vi "SciShutter.vi"(7 "Operational Mode":T1, 8 "error in (no error)":errorcluster, 11 "Science":T2={"Time Stamp Control"=timestamp(0 s since 1904-01-01), "State"=FALSE, "Set"=enum."Arm"}) -> (0 "error out":errorcluster={"status"=FALSE, "code"=180121602, "source"="Shared Variable in SciShutter.vi->MainRT.vi<APPEND>\nThis error or warning occurred while reading the following Shared Variable:\n\\\\.\\RT-Variables\\Dummy Trigger\n\\\\.\\RT-Variables\\Dummy Trigger"}, 3 "Science out":T2, 5 "Operational Mode out":T1)   [LabVIEW 2016]
uses:
  Controls/Shutter Data.ctl
  Controls/Shutter States.ctl
  Controls/Operational Modes.ctl
panel:
  in  "Wait time [s]":dbl=0.1 format="%#_13g"
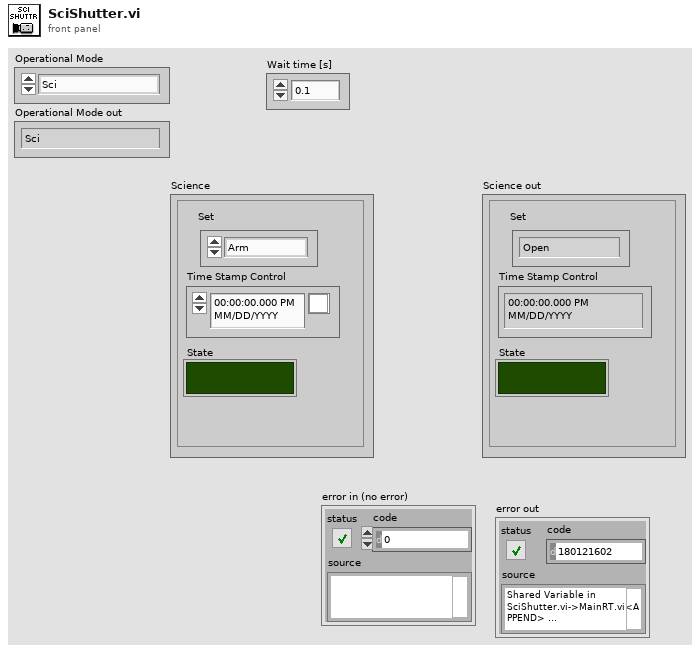
[diagram p1: front panel]
types:
  T1 = typedef "Operational Modes.ctl" = enum16{"Sci", "Sci-LFC", "Solar", "Solar-LFC", "LFC", "LFC-Sim", "LFC-Both", "ThAr", "ThAr-LFC", "Flat", "ExtFlat", "ExtFlat-Sim", "ExtFlat-Both", "Qtz", "ExtQtz", "ExtQtz-Sim", "ExtQtz-Both", "Dark", "Manual", "Off"}
  T2 = typedef "Shutter Data.ctl" = cluster{"Time Stamp Control":timestamp, "State":bool, "Set":T3}
  T3 = typedef "Shutter States.ctl" = enum16{"Open", "Close", "Wait", "Off", "Arm", "Idle"}
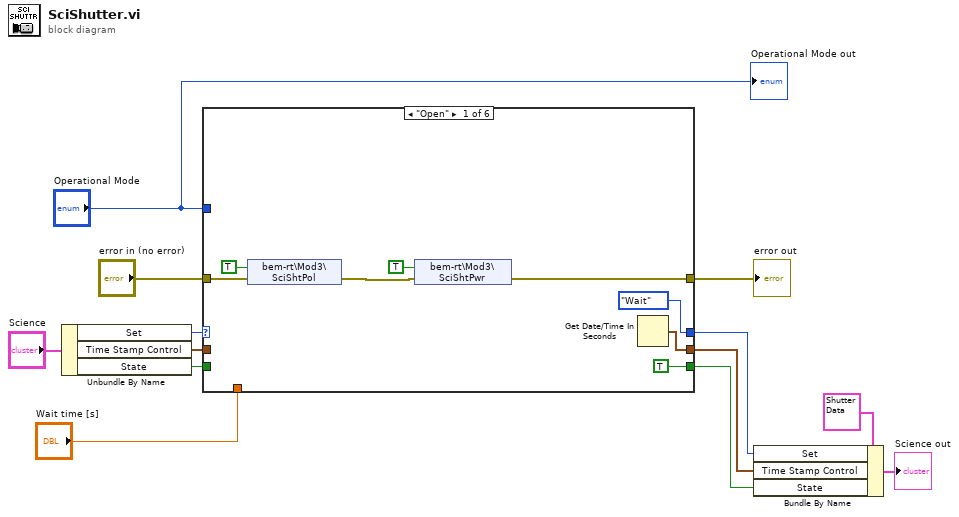
[diagram p0: block diagram]
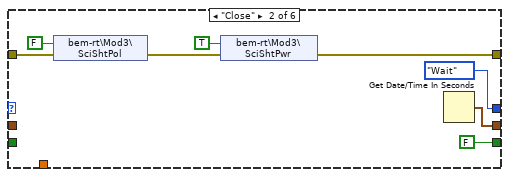
[diagram p2: hidden frame]
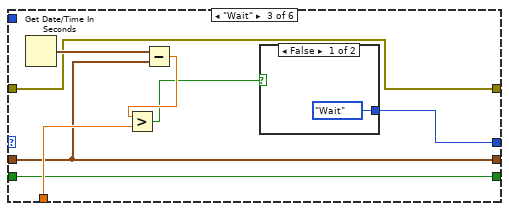
[diagram p3: hidden frame]
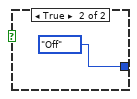
[diagram p4: hidden frame]
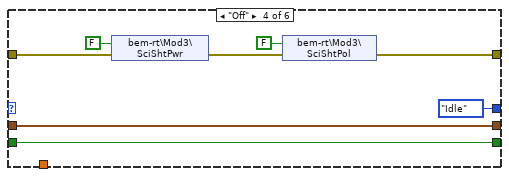
[diagram p5: hidden frame]
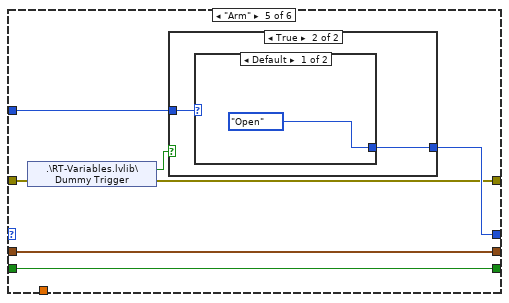
[diagram p6: hidden frame]
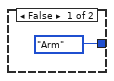
[diagram p7: hidden frame]
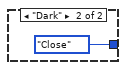
[diagram p8: hidden frame]
diagram:
  n1 = Unbundle By Name("Science") -> ("Set"=w13:T3, "Time Stamp Control"=w11:timestamp, "State"=w9:bool)
  n2 = case shown="\"Open\"" w13 {
    selector: w13 -> [_ _ _ _ _ w63]
    tunnel: [Shutter_States."Wait" ("Set") Shutter_States."Wait" ("Set") w33 Shutter_States."Idle" ("Set") w53 w63] -> w4
    tunnel: w11 -> [_ _ w32 w41 w49 w62]
    tunnel: [w21 w26 w32 w41 w49 w62] -> w10
    tunnel: w9 -> [_ _ w31 w40 w52 w61]
    tunnel: [TRUE ("State") FALSE ("State") w31 w40 w52 w61] -> w8
    tunnel: [w19 w28 w30 w43 w51 w60] -> w7
    tunnel: "error in (no error)" -> [w18 w27 w30 w45 w50 w60]
    tunnel: "Wait time [s]" -> [_ _ w35 _ _ _]
    tunnel: "Operational Mode" -> [_ _ _ _ w48 _]
    frame "Open" {
      n3 = shared-variable "bem-rt\\Mod3\\SciShtPol"(TRUE ("SciShtPol"), error in=w18) -> (error out=w17:errorcluster)
      n4 = shared-variable "bem-rt\\Mod3\\SciShtPwr"(TRUE ("SciShtPwr"), error in=w17) -> (error out=w19:errorcluster)
      n5 = Get Date/Time In Seconds() -> (seconds since 1Jan1904=w21:timestamp)
    }
    frame "Close" {
      n6 = shared-variable "bem-rt\\Mod3\\SciShtPol"(FALSE ("SciShtPol"), error in=w27) -> (error out=w29:errorcluster)
      n7 = shared-variable "bem-rt\\Mod3\\SciShtPwr"(TRUE ("SciShtPwr"), error in=w29) -> (error out=w28:errorcluster)
      n8 = Get Date/Time In Seconds() -> (seconds since 1Jan1904=w26:timestamp)
    }
    frame "Wait" {
      n9 = Get Date/Time In Seconds() -> (seconds since 1Jan1904=w37:timestamp)
      n10 = Subtract(x=w37, y=w32) -> (x-y=w36:dbl)
      n11 = Greater?(x=w36, y=w35) -> (0:w34:bool)
      n12 = case shown="False" w34 {
        tunnel: [Shutter_States."Wait" ("Set") Shutter_States."Off" ("Set")] -> w33
        frame False {
        }
        frame True {
        }
      }
    }
    frame "Off" {
      n13 = shared-variable "bem-rt\\Mod3\\SciShtPwr"(FALSE ("SciShtPwr"), error in=w45) -> (error out=w44:errorcluster)
      n14 = shared-variable "bem-rt\\Mod3\\SciShtPol"(FALSE ("SciShtPol"), error in=w44) -> (error out=w43:errorcluster)
    }
    frame "Arm" {
      n15 = shared-variable ".\\RT-Variables.lvlib\\Dummy Trigger"(error in=w50) -> (w54:bool, error out=w51:errorcluster)
      n16 = case shown="True" w54 {
        tunnel: [Shutter_States."Arm" ("Set") w57] -> w53
        tunnel: w48 -> [_ w56]
        frame False {
        }
        frame True {
          n17 = case shown="Default" w56 {
            tunnel: [Shutter_States."Open" ("Set") Shutter_States."Close" ("Set")] -> w57
            frame Default {
            }
            frame "Dark" {
            }
          }
        }
      }
    }
    frame "Idle" {
    }
  }
  "error out" <- w7
  n18 = Bundle By Name(cluster=T2 {"Time Stamp Control"=timestamp(0 s since 1904-01-01), "State"=FALSE, "Set"=enum."Open"} ("Shutter"), "Set"=w4, "Time Stamp Control"=w10, "State"=w8) -> (→"Science out":T2)
  "Operational Mode out" <- "Operational Mode"
